vi "Voltage - Finite Output.vi"() -> ()   [LabVIEW 2015]
doc: "This example demonstrates how to generate a finite amount of data from a buffer in your computer's memory."
uses:
  <vilib>/Utility/error.llb/DialogType.ctl
  <vilib>/DAQmx/write.llb/DAQmx Write (Analog Wfm 1Chan NSamp).vi
  <vilib>/DAQmx/create/channels.llb/DAQmx Create Channel (AO-Voltage-Basic).vi
  <vilib>/Utility/file.llb/Read Delimited Spreadsheet (DBL).vi
  <vilib>/DAQmx/configure/timing.llb/DAQmx Timing (Use Waveform).vi
  <vilib>/DAQmx/configure/trigger.llb/DAQmx Start Trigger (Digital Edge).vi
  <vilib>/DAQmx/configure/trigger.llb/DAQmx Start Trigger (Analog Edge).vi
  <vilib>/DAQmx/miscellaneous.llb/DAQmx Fill In Error Info.vi
  <resource>/objmgr/daqmx.rc
panel:
  in  "Scale Wave":dbl
  in  "maximum value":dbl=10.0 format="%0.2f"
  out "RMS":dbl
  out "Positive Peak":dbl
  out "Peak to Peak":dbl
  out "Negative Peak":dbl
  out "Samples":i32
  out "Path to EEG data":path
  in  "Trigger Type":T1(tab)
  in  "Edge":i32(ring)=10280 items=["Rising"=10280, "Falling"=10171]
  in  "Digital Trigger Source":tag
  in  "Level (V)":dbl format="%0.2f"
  in  "Hysteresis (V)":dbl
  in  "Slope":i32(ring)=10280 items=["Rising"=10280, "Falling"=10171]
  in  "Analog Trigger Source":string="APFI0"
  out "Waveform Graph":waveform(dbl)(graph)
  in  "Sample Rate":dbl=120000.0
  in  "Physical Channel(s)":tag="Dev1/ao0"
  out "Actual Sample Rate":dbl=1000.0 format="%0.2f"
  # "Channel Settings"
  # "Output"
  # "Signal info"
  # "Timing and Buffer Settings"
  # "Trigger Settings"
  # "Waveform Settings"
  # "default RMS is 1V\nbut signal rms was 15 uV"
  # "The number of elements in the waveform array must equal the number of channels in the task."
  # "To configure and use a start trigger you must have the necessary tab selected above.  Not all hardware supports triggering--refer to your device documentation for more info."
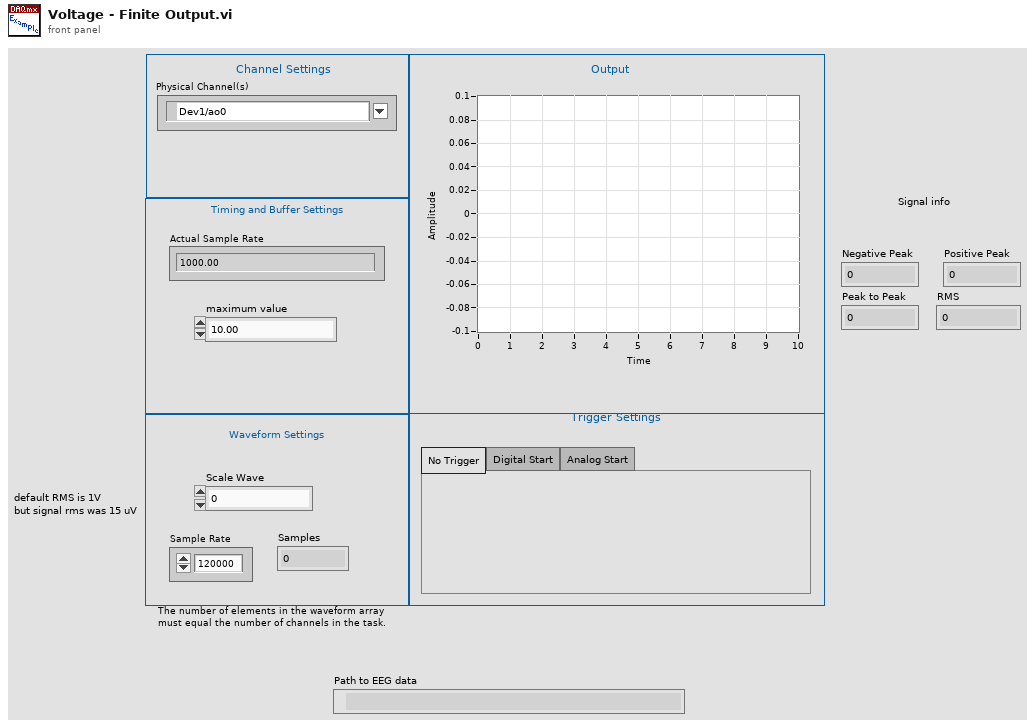
[diagram p1: front panel]
types:
  T1 = enum32{"No Trigger", "Digital Start", "Analog Start"}
  T2 = typedef "DialogType.ctl" = u16
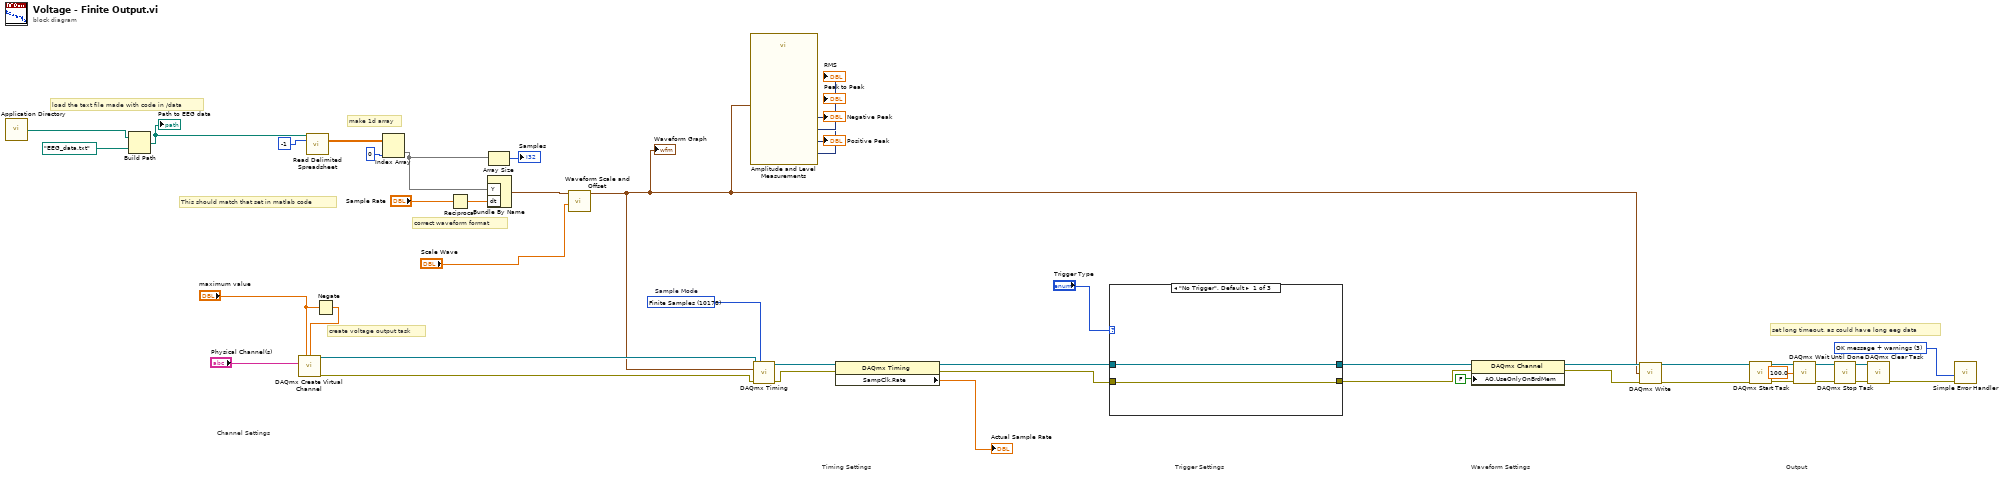
[diagram p0: block diagram]
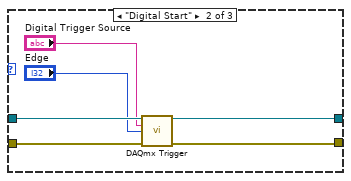
[diagram p2: hidden frame]
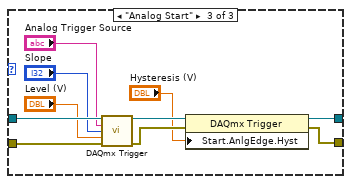
[diagram p3: hidden frame]
diagram:
  w27 = T2 3 items=["no dialog", "OK message", "continue or stop message", "OK message + warnings", "continue/stop + warnings"] ("type of dialog (OK msg:1)")
  w43 = 10178 items=["Finite Samples"=10178, "Continuous Samples"=10123, "Hardware Timed Single Point"=12522]  # Sample Mode
  # "set long timeout, as could have long eeg data"
  # "create voltage output task"
  # "correct waveform format"
  # "make 1d array"
  # "This should match that set in matlab code"
  # "load the text file made with code in /data"
  # "Output"
  # "Trigger Settings"
  # "Waveform Settings"
  # "Timing Settings"
  # "Channel Settings"
  n1 = call <vilib>:"Application Directory.vi"() -> ("Application Directory"=w16:path)
  n2 = Build Path(base path=w16, name or relative path=path "EEG_data.txt" ("file path (dialog if empty)")) -> (appended path=w17:path)
  "Path to EEG data" <- w17
  n3 = call-poly <vilib>:"Read Delimited Spreadsheet.vi"("file path (dialog if empty)"=w17, "number of rows (all:-1)"=-1) -> ("all rows"=w15:dbl[][])  [unwired: 8 in, 5 out]
  n4 = Negate(x="maximum value") -> (-x=w2:dbl)
  n5 = call-poly <vilib>:"DAQmx Create Virtual Channel.vi"("maximum value"="maximum value", "minimum value"=w2, "physical channels"="Physical Channel(s)") -> ("task out"=w42:refnum<k21>, "error out"=w10:errorcluster)  [unwired: 11 in]
  n6 = Index Array(array=w15, index (col)=0 ("disabled index (col)")) -> (element=w13:dbl[])  [unwired: 1 in]
  n7 = Reciprocal(x="Sample Rate") -> (1/x=w20:dbl)
  n8 = Bundle By Name("Y"=w13, "dt"=w20) -> (w5:waveform(dbl))  [unwired: 1 in]
  n9 = Array Size(array=w13) -> (size(s)=→"Samples":i32)
  n10 = call <vilib>:"Waveform Scale and Offset.vi"("scale"="Scale Wave", "waveform in"=w5) -> ("waveform out"=w4:waveform(dbl))  [unwired: 8 in, 1 out]
  "Waveform Graph" <- w4
  n11 = call "Amplitude and Level Measurements"("Signals"=w4) -> ("RMS"=→"RMS":dynamicdata, "Negative Peak"=→"Negative Peak":dynamicdata, "Positive Peak"=→"Positive Peak":dynamicdata, "Peak to Peak"=→"Peak to Peak":dynamicdata)  [unwired: 10 in, 1 out]
  n12 = call-poly <vilib>:"DAQmx Timing.vi"("task/channels in"=w42, "sample mode"=w43, "waveform"=w4, "error in"=w10) -> ("task out"=w45:refnum<k21>, "error out"=w44:errorcluster)  [unwired: 10 in]
  n13 = property class="DAQmx Timing"(reference=w45, error in=w44) -> (reference out=w38:refnum<k21>, error out=w37:errorcluster, "SampClk.Rate"=→"Actual Sample Rate":dbl)
  n14 = case shown="\"No Trigger\", Default" "Trigger Type" {
    tunnel: w38 -> [w47 w53 w63]
    tunnel: w37 -> [w46 w52 w62]
    tunnel: [w47 w51 w60] -> w23
    tunnel: [w46 w50 w59] -> w25
    frame "No Trigger", Default {
    }
    frame "Digital Start" {
      n15 = call-poly <vilib>:"DAQmx Trigger.vi"("task/channels in"=w53, "source"="Digital Trigger Source", "edge"="Edge", "error in"=w52) -> ("task out"=w51:refnum<k21>, "error out"=w50:errorcluster)  [unwired: 10 in]
    }
    frame "Analog Start" {
      n16 = call-poly <vilib>:"DAQmx Trigger.vi"("task/channels in"=w63, "source"="Analog Trigger Source", "slope"="Slope", "level"="Level (V)", "error in"=w62) -> ("task out"=w58:refnum<k21>, "error out"=w57:errorcluster)  [unwired: 9 in]
      n17 = property class="DAQmx Trigger"(reference=w58, error in=w57, "Start.AnlgEdge.Hyst"="Hysteresis (V)") -> (reference out=w60:refnum<k21>, error out=w59:errorcluster)
    }
  }
  n18 = property class="DAQmx Channel"(reference=w23, error in=w25, "AO.UseOnlyOnBrdMem"=FALSE) -> (reference out=w22:refnum<k21>, error out=w24:errorcluster)
  n19 = call-poly <vilib>:"DAQmx Write.vi"("task/channels in"=w22, "data"=w4, "error in"=w24) -> ("task out"=w36:refnum<k21>, "error out"=w35:errorcluster)  [unwired: 10 in, 1 out]
  n20 = call <vilib>:"DAQmx Start Task.vi"("task/channels in"=w36, "error in"=w35) -> ("task out"=w34:refnum<k21>, "error out"=w33:errorcluster)  [unwired: 12 in]
  n21 = call <vilib>:"DAQmx Wait Until Done.vi"("task/channels in"=w34, "timeout (sec)"=100.0, "error in"=w33) -> ("task out"=w29:refnum<k21>, "error out"=w28:errorcluster)  [unwired: 11 in]
  n22 = call <vilib>:"DAQmx Stop Task.vi"("task/channels in"=w29, "error in"=w28) -> ("task out"=w31:refnum<k21>, "error out"=w30:errorcluster)  [unwired: 12 in]
  n23 = call <vilib>:"DAQmx Clear Task.vi"("task in"=w31, "error in"=w30) -> ("error out"=w41:errorcluster)  [unwired: 13 in]
  n24 = call <vilib>:"Simple Error Handler.vi"("type of dialog (OK msg:1)"=w27, "error in (no error)"=w41) -> ()  [unwired: 3 in, 5 out]
